vi "Push Element.vi"(8 "error in":errorcluster, 10 "element":variant, 11 "Buffer in":refnum<data-value>) -> (0 "error out":errorcluster, 3 "Buffer":refnum<data-value>)   [LabVIEW 2013, in "VariantBuffer.lvclass"]
doc: "This VI writes one data element into the current location in the buffer. The location in the buffer is updated automatically."
uses:
  VariantBuffer.lvclass
  VariantBuffer.lvclass/VariantBuffer.ctl
panel:
  out "overflowed?":bool
  out "overflow":variant
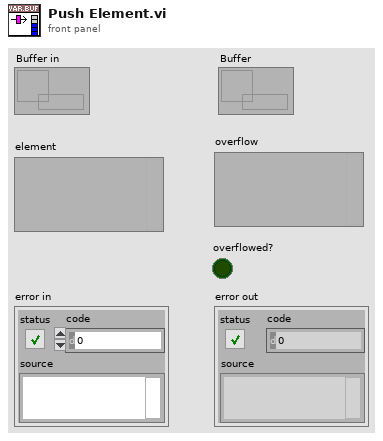
[diagram p1: front panel]
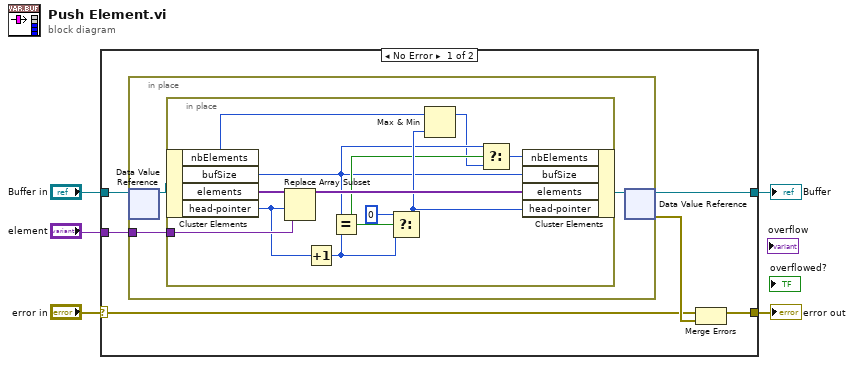
[diagram p0: block diagram]
diagram:
  n1 = case shown="No Error" "error in" {
    selector: "error in" -> [w6 w28]
    tunnel: "Buffer in" -> [w11 w27]
    tunnel: [w10 w27] -> w4
    tunnel: [w8 w28] -> w3
    tunnel: "element" -> [w7 _]
    frame No Error {
      n2 = in-place {
        in-place-border: w7 -> [w14]
        n3 = in-place-dvr #1(w11) -> (w13:refnum<class "VariantBuffer.lvclass">)  [unwired: 1 out]
        n4 = in-place {
          in-place-border: w14 -> [w23]
          n5 = in-place-cluster #2(w13) -> ("nbElements"=w21:i32, "bufSize"=w17:i32, "elements"=w26:variant[], "head-pointer"=w22:i32)
          n6 = Replace Array Subset(array=w26, new element=w23, index=w22) -> (w25:variant[])
          n7 = Increment(x=w22) -> (x+1=w20:i32)
          n8 = Equal?(x=w17, y=w20) -> (x = y?=w18:bool)
          n9 = Select(t=0, s=w18, f=w20) -> (s? t:f=w19:i32)
          n10 = Max & Min(x=w21, y=w19) -> (max(x,y)=w16:i32)  [unwired: 1 out]
          n11 = Select(t=w17, s=w18, f=w16) -> (s? t:f=w15:i32)
          n12 = in-place-cluster #2("nbElements"=w15, "bufSize"=w17, "elements"=w25, "head-pointer"=w19) -> (w12:refnum<class "VariantBuffer.lvclass">)
        }
        n13 = in-place-dvr #1(w12) -> (w10:refnum<data-value>, w9:errorcluster)
      }
      n14 = Merge Errors(w6, w9) -> (w8:errorcluster)
    }
    frame Error {
    }
  }
  "error out" <- w3
  "Buffer" <- w4
